vi "SwerveDriveRotate.vi"(0 "Strafe Joystick Axes":cluster{"X":dbl, "Y":dbl}, 1 "Center of Rotation Joystick Axes":cluster{"X":dbl, "Y":dbl}, 2 "Trigger Axes":cluster{"Left":dbl, "Right":dbl}, 4 "Angle (degrees; 0 = right)":dbl, 5 "error in (no error)":errorcluster, 6 "Strafe Multiplier":dbl, 7 "FieldCentric? (T)":bool=TRUE, 8 "Rotation Multiplier":dbl, 10 "Max Wheel Speed":dbl) -> (16 "Speed Chart":cluster{dbl, "Encoder Velocity":dbl}[](graph), 17 "Position Chart":cluster{dbl, "Encoder Velocity":dbl}[](graph), 19 "error out":errorcluster)   [LabVIEW 2014, in "Team900SwerveDrive.lvlib"]
uses:
  Team900SwerveDrive.lvlib
  <vilib>/Rock Robotics/WPI/CAN/TalonSRX/WPI_CANTalonSRX_APIControlMode.ctl
  <vilib>/Rock Robotics/Network Tables/NT Write Numeric Array.vi
  Team900-VIs/Logitech/F510/F510-X.vi
panel:
  in  "Speed PID":cluster{"P":dbl, "I":dbl, "D":dbl}={"P"=0.0275, "I"=0.000115, "D"=0.682955}
  in  "Speed PID 2":cluster{"P":dbl, "I":dbl, "D":dbl}={"P"=0.0275, "I"=0.000115, "D"=0.682955}
  in  "% VBus":dbl
  # "Most basic version of SwerveDrive, expects two joystick inputs, one for\nstrafe, one for the center of rotation (can be left unwired if you just\nwant the robot to rotate around its center), and triggers for rotation\n(pressing the right trigger rotates clockwise, left trigger counterclockwise)\n\nIf the FieldCentric control is false, then up on the joystick is forward for the\nrobot; if it is true then the strafe vector is rotated based on the Angle input\nso that up on the strafe joystick drives in a constant direction regardless\nof robot heading."
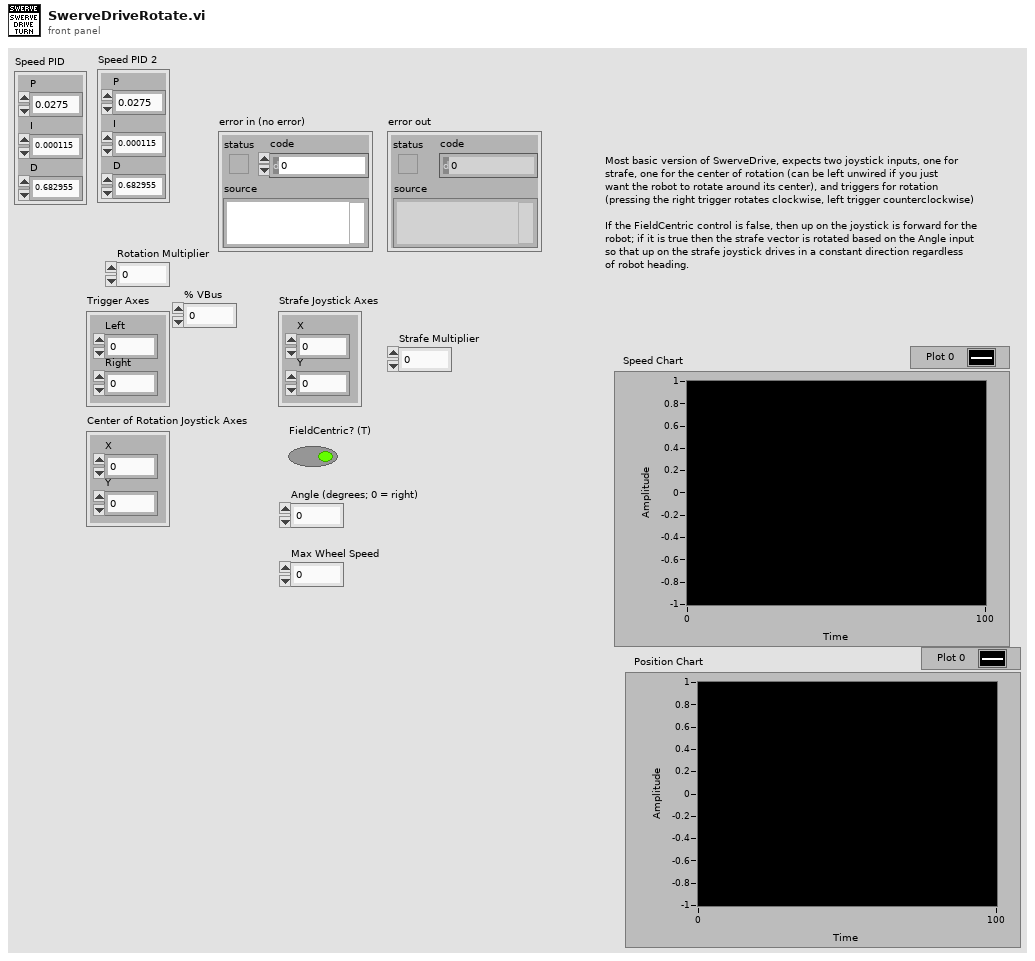
[diagram p1: front panel]
types:
  T1 = cluster{"Up":bool, "Right":bool, "Down":bool, "Left":bool}
  T2 = typedef "WPI_CANTalonSRX_APIControlMode.ctl" = enum8{"Percent VBus", "Speed", "Position", "Slave", "Unchanged / Invalid"}
  T3 = typedef "WPI_MotorControlDeviceRef.ctl" = cluster{"DeviceStatus":errorcluster, "Type":T4, "PWM":cluster{"Controller":T5, "PWM Channel":T6, "DeadBand":T7}, "CAN":cluster{"Device Number":u8, "Control Mode":T8, "Semaphore":T9, "Max Vout":dbl, "TalonSRX Control Mode":T2}, "Invert":bool, "TransformRef":T10, "InvTransformRef":T10}
  T4 = typedef "WPI_MotorControlType.ctl" = enum16{"PWM", "CAN", "CANTalonSRX"}
  T5 = typedef "FPGA_TypedefDigitalModule.ctl" = enum16{"Controller 1"}
  T6 = typedef "FPGA_DIOPWMChannel.ctl" = enum8{"PWM 0", "PWM 1", "PWM 2", "PWM 3", "PWM 4", "PWM 5", "PWM 6", "PWM 7", "PWM 8", "PWM 9", "PWM MXP 0", "PWM MXP 1", "PWM MXP 2", "PWM MXP 3", "PWM MXP 4", "PWM MXP 5", "PWM MXP 6", "PWM MXP 7", "PWM MXP 8", "PWM MXP 9", "Invalid"}
  T7 = typedef "WPI_PWMDeadband.ctl" = cluster{"Name":string, "maxPositivePwm":i32, "minPositivePwm":i32, "centerPwm":i32, "maxNegativePwm":i32, "minNegativePwm":i32, "angularRange":u16}
  T8 = typedef "WPI_CANJaguar_ControlMode.ctl" = enum8{"Percent VBus", "Current", "Speed", "Position", "Voltage"}
  T9 = typedef "Semaphore RefNum" = refnum<k1>
  T10 = typedef "WPI_PWMTransform_ConPane.ctl" = refnum<vi>
  T11 = cluster{"FL Speed":T3, "FR Speed":T3, "RL Speed":T3, "RR Speed":T3}
  T12 = cluster{"FL Steering":T3, "FR Steering":T3, "RL Steering":T3, "RR Steering":T3}
  T13 = typedef "WPI_CANTalonSRX_GlobalStatus.ctl" = cluster{"Applied Throttle":dbl, "Module Enabled":bool, "CAN Error":errorcluster, "Closed Loop Error":dbl, "Forward Limit Switch Closed":bool, "Reverse Limit Switch Closed":bool, "Sensor Position":dbl, "Sensor Velocity":dbl, "Current":dbl, "Sticky Fault - Over Temp":bool, "Sticky Fault - Under Voltage":bool, "Sticky Fault - Forward Limit":bool, "Sticky Fault - Reverse Limit":bool, "Sticky Fault - Forward Soft Limit":bool, "Sticky Fault - Reverse Soft Limit":bool, "Brake is Enabled":bool, "Encoder Position":dbl, "Encoder Velocity":dbl, "Encoder Index Count":dbl, "Encoder A Pin State":bool, "Encoder B Pin State":bool, "Encoder Index Pin State":bool, "Analog In":dbl, "Analog In Velocity":dbl, "Temperature (C)":dbl, "Battery Voltage":dbl}
  T14 = cluster{"output angle":dbl, "Encoder Velocity":dbl}
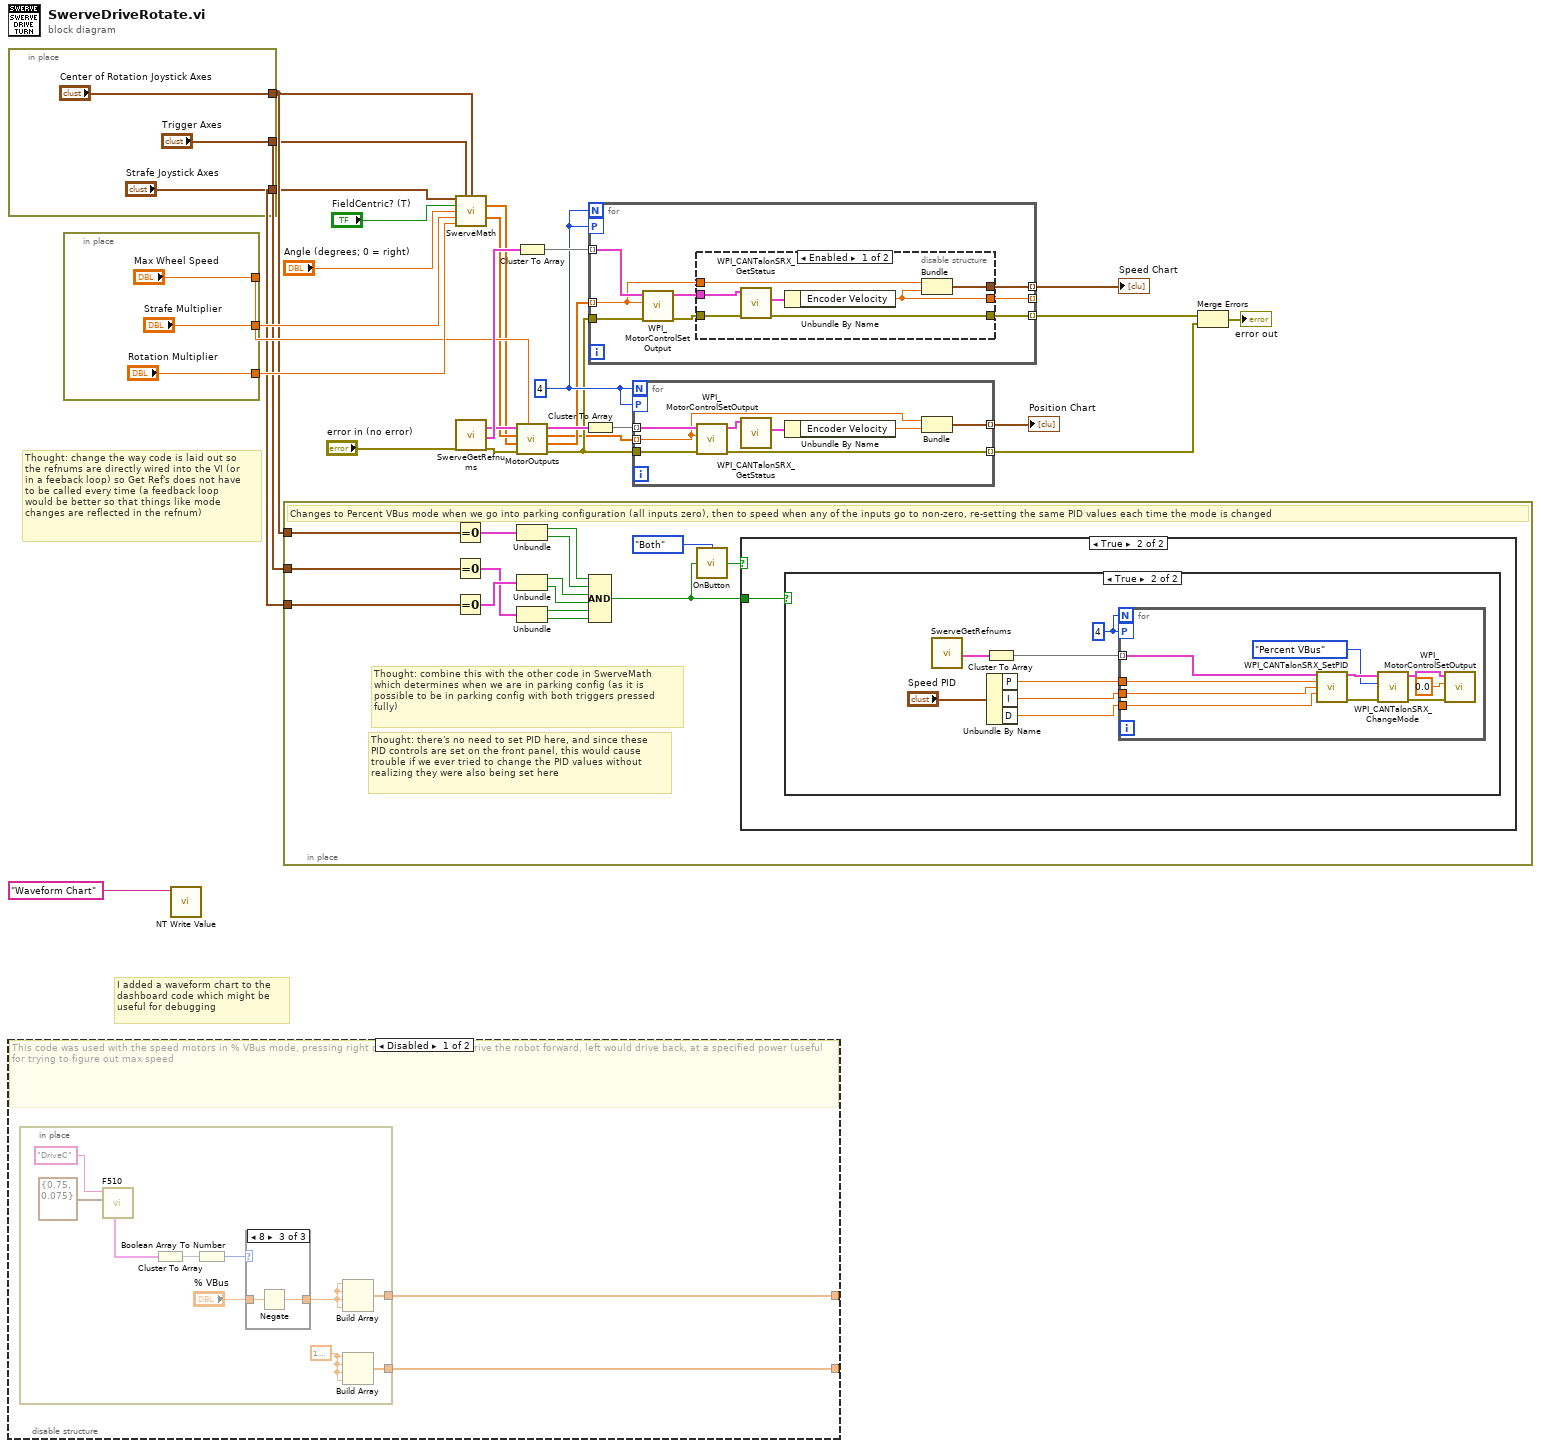
[diagram p0: block diagram]
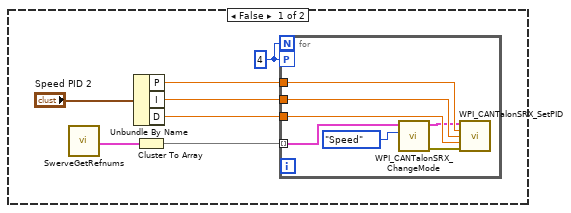
[diagram p3: hidden frame]
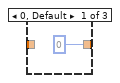
[diagram p4: hidden frame]
diagram:
  w17 = 4
  # "Thought: change the way code is laid out so\nthe refnums are directly wired into the VI (or\nin a feeback loop) so Get Ref's does not have\nto be called every time (a feedback loop\nwould be better so that things like mode \nchanges are reflected in the refnum)"
  # "I added a waveform chart to the\ndashboard code which might be\nuseful for debugging"
  n1 = in-place {
    in-place-border: ["Center of Rotation Joystick Axes"] -> w3
    in-place-border: ["Strafe Joystick Axes"] -> w2
    in-place-border: ["Trigger Axes"] -> w1
  }
  n2 = disable-structure shown="Disabled" {
    disable-tunnel: [w32 _] -> _
    disable-tunnel: [w31 _] -> _
    frame Disabled {
      # "This code was used with the speed motors in % VBus mode, pressing right on the D-pad would drive the robot forward, left would drive back, at a specified power (useful for trying to figure out max speed"
      n3 = in-place {
        in-place-border: [w40] -> w32
        in-place-border: [w38] -> w31
        w39 = 1.5707963267948966
        n4 = call-poly "F510.vi"("Deadzone Scale Cluster"=cluster{"Scale":dbl, "Deadzone":dbl} {"Scale"=0.75, "Deadzone"=0.075}, "refnum name"="DriveC") -> ("D-Pad Buttons"=w36:T1)  [unwired: 3 in, 6 out]
        n5 = Cluster To Array(cluster=w36) -> (array=w37:bool[])
        n6 = Boolean Array To Number(Boolean array=w37) -> (number=w35:u32)
        n7 = case shown="8" w35 {
          tunnel: "% VBus" -> [_ w44 w46]
          tunnel: [0 w44 w45] -> w34
          frame 0, Default {
          }
          frame 2 {
          }
          frame 8 {
            n8 = Negate(x=w46) -> (-x=w45:dbl)
          }
        }
        n9 = Build Array(w34, w34, w34, w34) -> (w40:dbl[])
        n10 = Build Array(w39, w39, w39, w39) -> (w38:dbl[])
      }
    }
    frame Enabled {
    }
  }
  n11 = in-place {
    in-place-border: ["Max Wheel Speed"] -> w11
    in-place-border: ["Rotation Multiplier"] -> w20
    in-place-border: ["Strafe Multiplier"] -> w19
  }
  n12 = call-poly <vilib>:"NT Write Value.vi"("Name"="Waveform Chart") -> ()  [unwired: 10 in, 1 out]
  n13 = in-place {
    in-place-border: w3 -> [w52]
    in-place-border: w2 -> [w51]
    in-place-border: w1 -> [w50]
    # "Thought: there's no need to set PID here, and since these\nPID controls are set on the front panel, this would cause\ntrouble if we ever tried to change the PID values without\nrealizing they were also being set here"
    # "Thought: combine this with the other code in SwerveMath\nwhich determines when we are in parking config (as it is\npossible to be in parking config with both triggers pressed\nfully)"
    # "Changes to Percent VBus mode when we go into parking configuration (all inputs zero), then to speed when any of the inputs go to non-zero, re-setting the same PID values each time the mode is changed"
    n14 = Equal To 0?(x=w52) -> (x = 0?=w56:cluster{"X":bool, "Y":bool})
    n15 = Equal To 0?(x=w50) -> (x = 0?=w54:cluster{"Left":bool, "Right":bool})
    n16 = Equal To 0?(x=w51) -> (x = 0?=w55:cluster{"X":bool, "Y":bool})
    n17 = Unbundle(w56) -> ("X"=w60:bool, "Y"=w59:bool)
    n18 = Unbundle(w55) -> ("X"=w62:bool, "Y"=w61:bool)
    n19 = Unbundle(w54) -> ("Left"=w58:bool, "Right"=w57:bool)
    n20 = Compound Arithmetic op=AND(w60, w59, w62, w61, w58, w57) -> (w53:bool)
    n21 = call "OnButton.vi"("Button"=w53, "Mode"=enum16{"Press", "Release", "Both"}."Both") -> ("Value"=w64:bool)
    n22 = case shown="True" w64 {
      tunnel: w53 -> [_ w65]
      frame False {
      }
      frame True {
        n23 = case shown="True" w65 {
          frame False {
            w66 = 4
            n24 = call "SwerveGetRefnums.vi"() -> ("Speed"=w71:T11)  [unwired: 9 in, 10 out]
            n25 = Unbundle By Name("Speed PID 2") -> ("P"=w70:dbl, "I"=w69:dbl, "D"=w68:dbl)
            n26 = Cluster To Array(cluster=w71) -> (array=w72:T3[])
            n27 = for {
              N: w66 -> [_]
              workers-P: w66 -> [_]
              tunnel: w72 -> [w75] mode=indexing
              tunnel: w70 -> [w77]
              tunnel: w69 -> [w78]
              tunnel: w68 -> [w79]
              n28 = call <vilib>:"WPI_CANTalonSRX_ChangeMode.vi"("Control Mode"=WPI_CANTalonSRX_APIControlMode."Speed", "CAN Talon SRX Ref"=w75) -> ("error out"=w73:errorcluster, "CAN Talon SRX Ref Out"=w74:T3)  [unwired: 8 in]
              n29 = call <vilib>:"WPI_CANTalonSRX_SetPID.vi"("CAN Talon SRX Ref"=w74, "P"=w77, "I"=w78, "D"=w79, "error in (no error)"=w73) -> ()  [unwired: 9 in, 2 out]
            }
          }
          frame True {
            w80 = 4
            n30 = call "SwerveGetRefnums.vi"() -> ("Speed"=w85:T11)  [unwired: 9 in, 10 out]
            n31 = Cluster To Array(cluster=w85) -> (array=w86:T3[])
            n32 = Unbundle By Name("Speed PID") -> ("P"=w84:dbl, "I"=w83:dbl, "D"=w82:dbl)
            n33 = for {
              N: w80 -> [_]
              workers-P: w80 -> [_]
              tunnel: w86 -> [w96] mode=indexing
              tunnel: w84 -> [w93]
              tunnel: w83 -> [w94]
              tunnel: w82 -> [w95]
              n34 = call <vilib>:"WPI_CANTalonSRX_SetPID.vi"("CAN Talon SRX Ref"=w96, "P"=w93, "I"=w94, "D"=w95) -> ("CAN Talon SRX Ref Out"=w92:T3, "error out"=w91:errorcluster)  [unwired: 10 in]
              n35 = call <vilib>:"WPI_CANTalonSRX_ChangeMode.vi"("error in (no error)"=w91, "Control Mode"=WPI_CANTalonSRX_APIControlMode."Percent VBus", "CAN Talon SRX Ref"=w92) -> ("error out"=w89:errorcluster, "CAN Talon SRX Ref Out"=w88:T3)  [unwired: 7 in]
              n36 = call <vilib>:"WPI_MotorControlSetOutput.vi"("error in (no error)"=w89, "Output"=0.0, "MotorControlDevRef"=w88) -> ()  [unwired: 6 in, 3 out]
            }
          }
        }
      }
    }
  }
  n37 = call "SwerveMath.vi"("Strafe Joystick Axes"=w2, "Trigger Axes"=w1, "Center of Rotation Joystick"=w3, "FieldCentric? (T)"="FieldCentric? (T)", "Angle (degrees; 0 = right)"="Angle (degrees; 0 = right)", "Strafe Multiplier"=w19, "Rotation Multiplier"=w20) -> ("Motor Speeds"=w8:dbl[], "Motor Angles"=w9:dbl[])  [unwired: 7 in]
  n38 = call "SwerveGetRefnums.vi"("error in (no error)"="error in (no error)") -> ("Steering"=w18:T12, "Speed"=w24:T11, "error out"=w14:errorcluster)  [unwired: 8 in, 8 out]
  n39 = Cluster To Array(cluster=w24) -> (array=w22:T3[])
  n40 = call "MotorOutputs.vi"("Max Wheel Speed"=w11, "error in (no error)"=w14, "Motor Speeds"=w8, "Target Angles"=w9, "Steering Refnums In"=w18) -> ("error out"=w13:errorcluster, "Speed Motor Setpoints"=w12:dbl[], "Steering Motor Setpoints"=w7:dbl[], "Steering Refnums Out"=w16:T12)  [unwired: 3 in]
  n41 = Cluster To Array(cluster=w16) -> (array=w15:T3[])
  n42 = for {
    N: w17 -> [_]
    tunnel: w13 -> [w104]
    tunnel: [w101] -> w23 mode=indexing
    workers-P: w17 -> [_]
    tunnel: w22 -> [w103] mode=indexing
    tunnel: [w99] -> _ mode=indexing
    tunnel: [w98] -> w5 mode=indexing
    tunnel: w12 -> [w97] mode=indexing
    n43 = call <vilib>:"WPI_MotorControlSetOutput.vi"("error in (no error)"=w104, "Output"=w97, "MotorControlDevRef"=w103) -> ("error out"=w102:errorcluster, "MotorControlDevRef"=w100:T3)  [unwired: 6 in, 1 out]
    n44 = disable-structure shown="Enabled" {
      disable-tunnel: w102 -> [w111 w112]
      disable-tunnel: [w110 w112] -> w101
      disable-tunnel: w100 -> [w109 _]
      disable-tunnel: [w107 _] -> w99
      disable-tunnel: [w105 _] -> w98
      disable-tunnel: w97 -> [w106 _]
      frame Enabled {
        n45 = call <vilib>:"WPI_CANTalonSRX_GetStatus.vi"("error in (no error)"=w111, "CAN Talon SRX Ref"=w109) -> ("error out"=w110:errorcluster, "Talon SRX Status"=w108:T13)  [unwired: 7 in, 1 out]
        n46 = Unbundle By Name(w108) -> ("Encoder Velocity"=w107:dbl)
        n47 = Bundle(w106, "Encoder Velocity"=w107) -> (w105:cluster{dbl, "Encoder Velocity":dbl})  [unwired: 1 in]
      }
      frame Disabled {
      }
    }
  }
  "Speed Chart" <- w5
  n48 = for {
    N: w17 -> [_]
    tunnel: w13 -> [w120]
    workers-P: w17 -> [_]
    tunnel: w15 -> [w119] mode=indexing
    tunnel: w7 -> [w114] mode=indexing
    tunnel: [w118] -> w10 mode=indexing
    tunnel: [w113] -> w4 mode=indexing
    n49 = call <vilib>:"WPI_MotorControlSetOutput.vi"("error in (no error)"=w120, "Output"=w114, "MotorControlDevRef"=w119) -> ("error out"=w118:errorcluster, "MotorControlDevRef"=w116:T3)  [unwired: 6 in, 1 out]
    n50 = call <vilib>:"WPI_CANTalonSRX_GetStatus.vi"("CAN Talon SRX Ref"=w116) -> ("Talon SRX Status"=w117:T13)  [unwired: 8 in, 2 out]
    n51 = Unbundle By Name(w117) -> ("Encoder Velocity"=w115:dbl)
    n52 = Bundle("output angle"=w114, "Encoder Velocity"=w115) -> (w113:T14)  [unwired: 1 in]
  }
  "Position Chart" <- w4
  n53 = Merge Errors(w23, w10) -> (→"error out":errorcluster)
